vi "2182Delta_LV6.vi"() -> ()   [LabVIEW 2022 SP3]
panel:
  out "Resistance of DUT":dbl[](graph)
  out "Resistance (m-Ohms)":dbl[](array[numeric]) format="%.10f"
  in  "Sample Count To Display":i32=10
  in  "2400 Trig Count":string="20"
  out "Voltage Drop Across DUT":dbl[](graph)
  out "Delta Readings (uV)":ext[](array[numeric]) format="%.12f"
  in  "2182 Buffer Points":string="10"
  in  "2400 CURR LIST":string="20E-6,-20E-6"
  in  "2400 GPIB add":string="24"
  in  "2182 GPIB add":string="25"
  # "KEITHLEY"
  # "Ultra Low Resistance - Delta Mode Measurements using 2400 and 2182."
  # "Connect Trigger Link Cable between 2182 & 2400.\nNote that moving average (digital) filter is on by default,\navg = 10rdgs, window = 0.01%"
  # "Note: If you change 2182 Buffer points you must also change 2400 Trigger count to \n2 x 2182 buffer points. You should also set the Sample count to display = 2182 Buffer Points.\nAlso change R=V/I calculation if you use different current!"
  # "Note: Change R=V/I in the program, if you change current!"
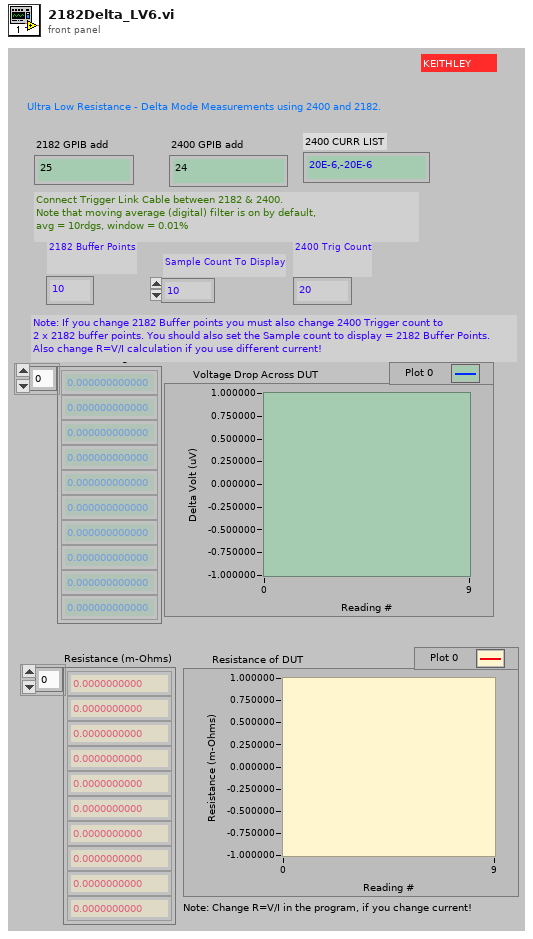
[diagram p1: front panel]
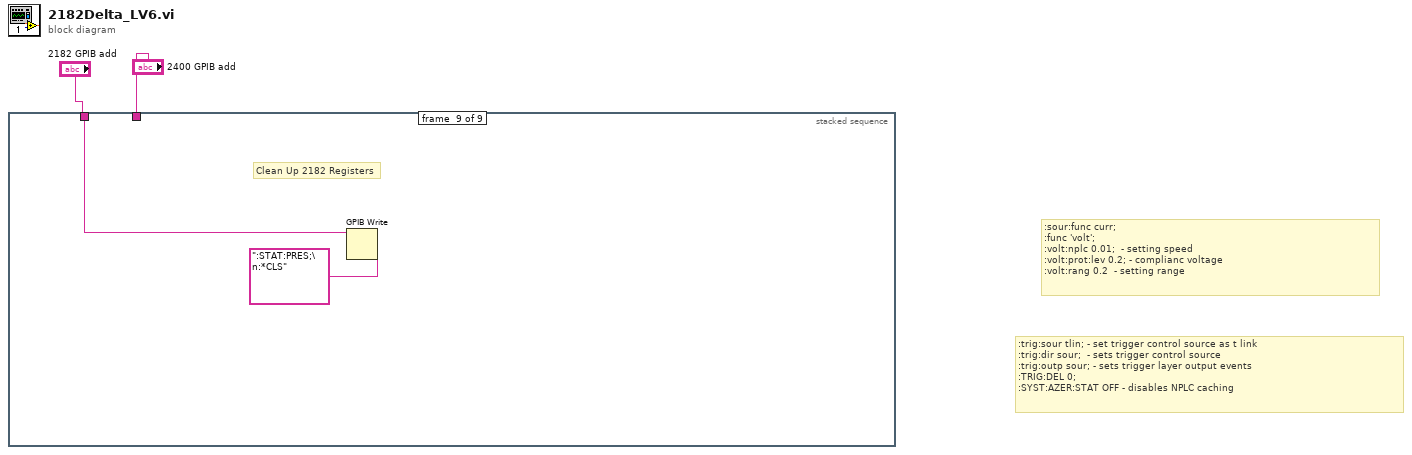
[diagram p0: block diagram]
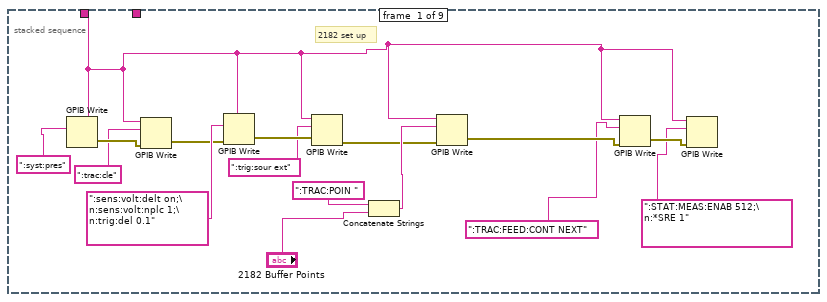
[diagram p2: hidden frame]
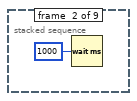
[diagram p3: hidden frame]
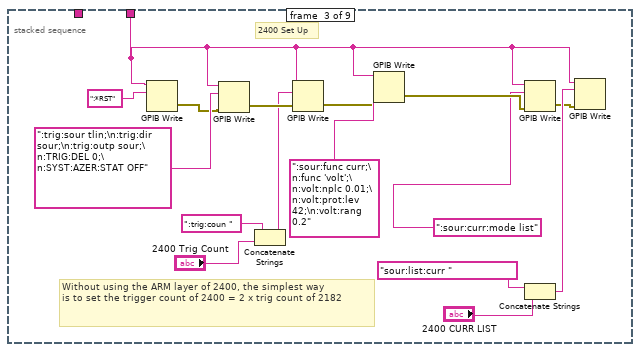
[diagram p4: hidden frame]
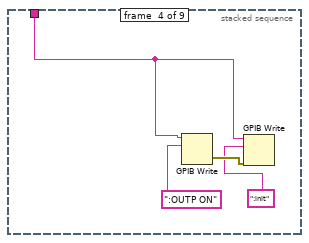
[diagram p5: hidden frame]
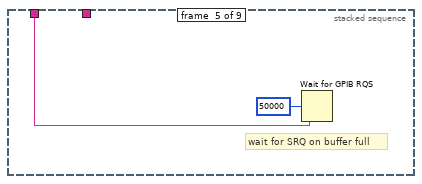
[diagram p6: hidden frame]
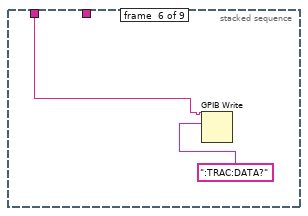
[diagram p7: hidden frame]
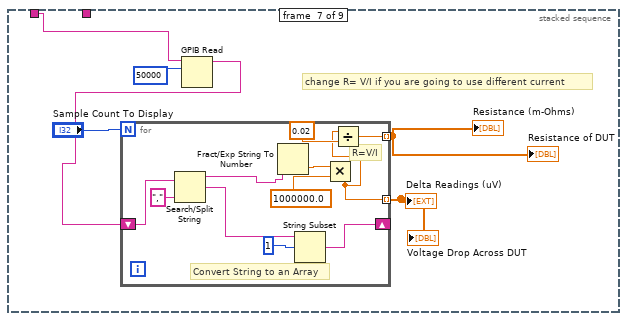
[diagram p8: hidden frame]
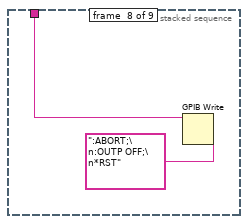
[diagram p9: hidden frame]
diagram:
  # ":trig:sour tlin; - set trigger control source as t link\n:trig:dir sour;  - sets trigger control source\n:trig:outp sour; - sets trigger layer output events\n:TRIG:DEL 0; \n:SYST:AZER:STAT OFF - disables NPLC caching"
  # ":sour:func curr;\n:func 'volt';\n:volt:nplc 0.01;  - setting speed\n:volt:prot:lev 0.2; - complianc voltage\n:volt:rang 0.2  - setting range"
  n1 = stacked-sequence {
    tunnel: "2182 GPIB add" -> [w6 _ _ _ w40 w42 w48 _ w63]
    tunnel: "2400 GPIB add" -> [_ _ w26 w36 _ _ _ w61 _]
    frame #0 {
      # "2182 set up"
      n2 = GPIB Write(0:w6, 1:":syst:pres") -> (6:w18:errorcluster)  [unwired: 3 in, 1 out]
      n3 = GPIB Write(0:w6, 1:":trac:cle", 3:w18) -> (6:w5:errorcluster)  [unwired: 2 in, 1 out]
      n4 = GPIB Write(0:w6, 1:":sens:volt:delt on;\n:sens:volt:nplc 1;\n:trig:del 0.1", 3:w5) -> (6:w9:errorcluster)  [unwired: 2 in, 1 out]
      n5 = GPIB Write(0:w6, 1:":trig:sour ext", 3:w9) -> (6:w4:errorcluster)  [unwired: 2 in, 1 out]
      n6 = Concatenate Strings(":TRAC:POIN ", "2182 Buffer Points") -> (w10:string)
      n7 = GPIB Write(0:w6, 1:w10, 3:w4) -> (6:w13:errorcluster)  [unwired: 2 in, 1 out]
      n8 = GPIB Write(0:w6, 1:":TRAC:FEED:CONT NEXT", 3:w13) -> (6:w15:errorcluster)  [unwired: 2 in, 1 out]
      n9 = GPIB Write(0:w6, 1:":STAT:MEAS:ENAB 512;\n:*SRE 1", 3:w15) -> ()  [unwired: 2 in, 2 out]
    }
    frame #1 {
      n10 = Wait (ms)(milliseconds to wait=u32 1000) -> ()  [unwired: 1 out]
    }
    frame #2 {
      # "Without using the ARM layer of 2400, the simplest way\nis to set the trigger count of 2400 = 2 x trig count of 2182"
      # "2400 Set Up"
      n11 = GPIB Write(0:w26, 1:":*RST") -> (6:w25:errorcluster)  [unwired: 3 in, 1 out]
      n12 = GPIB Write(0:w26, 1:":trig:sour tlin;\n:trig:dir sour;\n:trig:outp sour;\n:TRIG:DEL 0;\n:SYST:AZER:STAT OFF", 3:w25) -> (6:w24:errorcluster)  [unwired: 2 in, 1 out]
      n13 = Concatenate Strings(":trig:coun ", "2400 Trig Count") -> (w22:string)
      n14 = GPIB Write(0:w26, 1:w22, 3:w24) -> (6:w23:errorcluster)  [unwired: 2 in, 1 out]
      n15 = GPIB Write(0:w26, 1:":sour:func curr;\n:func 'volt';\n:volt:nplc 0.01;\n:volt:prot:lev 42;\n:volt:rang 0.2", 3:w23) -> (6:w30:errorcluster)  [unwired: 2 in, 1 out]
      n16 = GPIB Write(0:w26, 1:":sour:curr:mode list", 3:w30) -> (6:w31:errorcluster)  [unwired: 2 in, 1 out]
      n17 = Concatenate Strings("sour:list:curr ", "2400 CURR LIST") -> (w34:string)
      n18 = GPIB Write(0:w26, 1:w34, 3:w31) -> ()  [unwired: 2 in, 2 out]
    }
    frame #3 {
      n19 = GPIB Write(0:w36, 1:":OUTP ON") -> (6:w39:errorcluster)  [unwired: 3 in, 1 out]
      n20 = GPIB Write(0:w36, 1:":init", 3:w39) -> ()  [unwired: 2 in, 2 out]
    }
    frame #4 {
      # "wait for SRQ on buffer full"
      n21 = Wait for GPIB RQS(3:50000 ("timeout ms (488.2 global)"), 4:w40) -> ()  [unwired: 1 in, 2 out]
    }
    frame #5 {
      n22 = GPIB Write(0:w42, 1:":TRAC:DATA?") -> ()  [unwired: 3 in, 2 out]
    }
    frame #6 {
      # "change R= V/I if you are going to use different current"
      n23 = GPIB Read(0:w48, 1:50000 ("byte count")) -> (5:w46:string)  [unwired: 3 in, 2 out]
      n24 = for {
        N: "Sample Count To Display" -> [_]
        tunnel: [w51] -> w45 mode=indexing
        shift-right: [w56] -> _
        shift-left: w46 -> [w57]
        tunnel: [w53] -> w44 mode=indexing
        # "R=V/I"
        # "Convert String to an Array"
        n25 = Search/Split String(string=w57, search string/char (-)=",") -> (substring before match=w59:string, match + rest of string=w58:string)  [unwired: 1 in, 1 out]
        n26 = Fract/Exp String To Number(string=w59) -> (number=w50:dbl)  [unwired: 3 in, 1 out]
        n27 = String Subset(string=w58, offset (0)=1) -> (substring=w56:string)  [unwired: 1 in]
        n28 = Multiply(x=w50, y=1000000.0) -> (x*y=w51:dbl)
        n29 = Divide(x=w51, y=0.02 ("x")) -> (x/y=w53:dbl)
      }
      "Delta Readings (uV)" <- w45
      "Voltage Drop Across DUT" <- w45
      "Resistance (m-Ohms)" <- w44
      "Resistance of DUT" <- w44
    }
    frame #7 {
      n30 = GPIB Write(0:w61, 1:":ABORT;\n:OUTP OFF;\n*RST" ("data")) -> ()  [unwired: 3 in, 2 out]
    }
    frame #8 {
      # "Clean Up 2182 Registers"
      n31 = GPIB Write(0:w63, 1:":STAT:PRES;\n:*CLS" ("data")) -> ()  [unwired: 3 in, 2 out]
    }
  }
